vi "navX Open Serial.vi"(8 "error in (no error)":errorcluster, 9 "Raw Data":bool, 10 "Serial Port":T3, 11 "Update Rate (4Hz-60Hz)":u8) -> (0 "error out":errorcluster, 3 "navX Device":T1={"Interface"={"Protocol"=enum."SERIAL", "Update Rate (4Hz-60Hz)"=4, "navX Open TypeDef"=variant}, "Notify Packet"=refnum, "Loop VI Refnum"=refnum} {"Interface"."Update Rate (4Hz-60Hz)" min=4 max=60 step=1})   [LabVIEW 2014, in "navX Library v2.lvlib"]
uses:
  navX Library v2.lvlib
  NI WPI/WPI_SerialPort_USB.ctl
  TypeDefs/navX Device TypeDef.ctl
  TypeDefs/navX Protocol TypeDef.ctl
  TypeDefs/navX Notify Packet TypeDef.ctl
  TypeDefs/navX Action TypeDef.ctl
  TypeDefs/navX Open TypeDefs/navX Serial Open TypeDef.ctl
  NI WPI/NI WPI Serial USB.lvlib
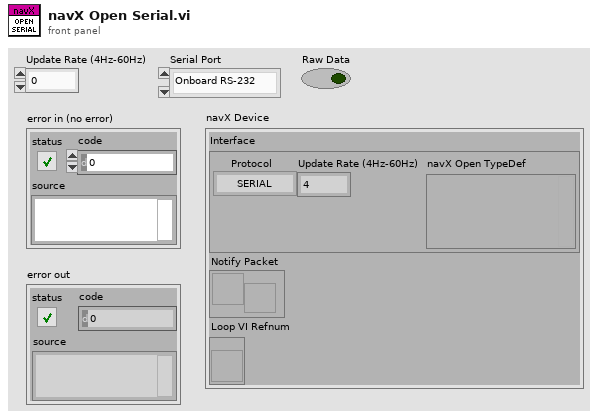
[diagram p1: front panel]
types:
  T1 = typedef "navX Library v2.lvlib/navX Device TypeDef.ctl" = cluster{"Interface":cluster{"Protocol":T2, "Update Rate (4Hz-60Hz)":u8, "navX Open TypeDef":variant}, "Notify Packet":refnum<notifier>, "Loop VI Refnum":refnum<vi>}
  T2 = typedef "navX Library v2.lvlib/navX Protocol TypeDef.ctl" = enum16{"SERIAL", "I2C", "SPI"}
  T3 = typedef "NI WPI Serial USB.lvlib/WPI_SerialPort_USB.ctl" = enum16{"Onboard RS-232", "MXP TTL", "USB"}
  T4 = typedef "navX Library v2.lvlib/navX Serial Open TypeDef.ctl" = cluster{"Serial Port":T3, "Raw Data":bool}
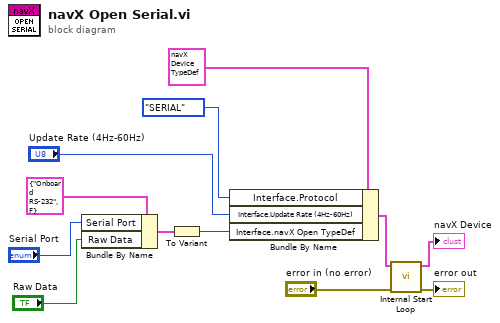
[diagram p0: block diagram]
diagram:
  n1 = Bundle By Name(cluster=T4 {"Serial Port"=enum."Onboard RS-232", "Raw Data"=FALSE} ("navX Serial Open"), "Serial Port"="Serial Port", "Raw Data"="Raw Data") -> (w11:T4)
  n2 = To Variant(anything=w11) -> (Variant=w9:variant)
  n3 = Bundle By Name(cluster=T1 {"Interface"={"Protocol"=enum."SERIAL", "Update Rate (4Hz-60Hz)"=4, "navX Open TypeDef"=variant}, "Notify Packet"=refnum, "Loop VI Refnum"=refnum} ("navX Device"), "Interface.Protocol"=navX_Protocol_TypeDef."SERIAL", "Interface.Update Rate (4Hz-60Hz)"="Update Rate (4Hz-60Hz)", "Interface.navX Open TypeDef"=w9) -> (w4:T1)
  n4 = call "Internal Start Loop.vi"("error in (no error)"="error in (no error)", "navX Device"=w4) -> ("error out"=→"error out":errorcluster, "navX Device"=→"navX Device":T1)  [unwired: 8 in]
